vi "FaceDL.vi"(0 "Data In":T8={"positions"=[1.0, 1.0, 1.0]} caption="Données en entrée", 2 "Display State In":T6={"param"=[], "positions"=[0.0, 0.0, 0.0], "CellsI"=enum."5", "CellsIII"=enum."7", "step,ps"=100, " preset pos"=[], "event"=refnum} caption="État d'affichage en entrée", 3 "Container State":T7 caption="État du conteneur") -> (6 "Data Out":T8={"positions"=[1.0, 1.0, 1.0]} caption="Données en sortie", 7 "Display State Out":T6={"param"=[], "positions"=[0.0, 0.0, 0.0], "CellsI"=enum."5", "CellsIII"=enum."7", "step,ps"=100, " preset pos"=[], "event"=refnum} caption="État d'affichage en sortie", 8 "Action":T5)   [LabVIEW 2020, in "ControlDL.xctl"]
uses:
  ControlDL.xctl
  DataDL.ctl
  <vilib>/_xctls/Container State.ctl
  stateDL.ctl
  controls/CellsSDI.ctl
  controls/CellBoolean.ctl
  controls/CellsSDIII.ctl
  <vilib>/_xctls/Action.ctl
  controls/DLSD.ctl
  controls/DLlongVerSD.ctl
  <vilib>/_xctls/XControlSupport.lvlib
panel:
  in  "CellsI":T1
  in  "param":cluster{"min":dbl, "max":dbl, "real pos":dbl}[](array[cluster])=[{"min"=-40.0, "max"=130.0, "real pos"=-130.0}, {"min"=-900.0, "max"=100.0, "real pos"=-100.0}, {"min"=-13.0, "max"=150.0, "real pos"=-137.0}]
  in  "posI":dbl caption="posI,mm"
  in  "DLI":T2=1.0 min=0.0 max=1.0 scale format="%#_6f"
  in  "step,ps":i32
  in  "Down":bool
  in  "Up":bool
  in  "posII":dbl caption="posII, mm"
  in  "DLII":T3=1.0 min=0.0 max=1.0 scale=-0.1..1.2 scale format="%.2f"
  in  "preset pos":dbl[][](array[numeric])=[[-48.0, -24.0, 0.0, 24.0, 48.0]]
  in  "CellsIII":T4=enum."1"
  in  "posIII":dbl
  in  "DLIII":T2=1.0 min=0.0 max=1.0 scale format="%#_6f"
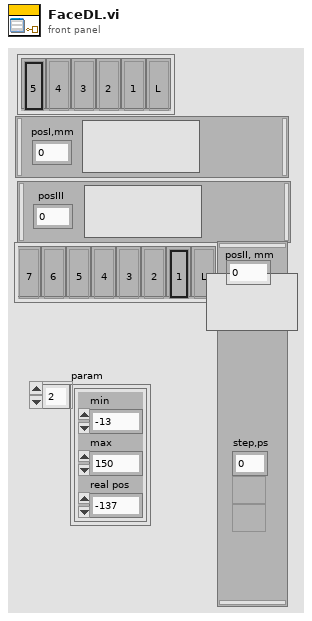
[diagram p1: front panel]
types:
  T1 = typedef "CellsSDI.ctl" = enum32{"5", "4", "3", "2", "1", "L"}
  T2 = typedef "DLSD.ctl" = dbl
  T3 = typedef "DLlongVerSD.ctl" = dbl
  T4 = typedef "CellsSDIII.ctl" = enum32{"7", "6", "5", "4", "3", "2", "1", "L"}
  T5 = typedef "XControlSupport.lvlib/Action.ctl" = cluster{"Data Changed?":bool, "State Changed?":bool, "Action Name":string}
  T6 = typedef "ControlDL.xctl/stateDL.ctl" = cluster{"param":cluster{"min":dbl, "max":dbl, "real pos":dbl}[], "positions":dbl[], "CellsI":T1, "CellsIII":T4, "step,ps":i32, " preset pos":dbl[][], "event":refnum<user-event>}
  T7 = typedef "XControlSupport.lvlib/Container State.ctl" = cluster{"Indicator?":bool, "Run Mode?":bool, " Refnum":refnum<vi>}
  T8 = typedef "ControlDL.xctl/DataDL.ctl" = cluster{"positions":dbl[]}
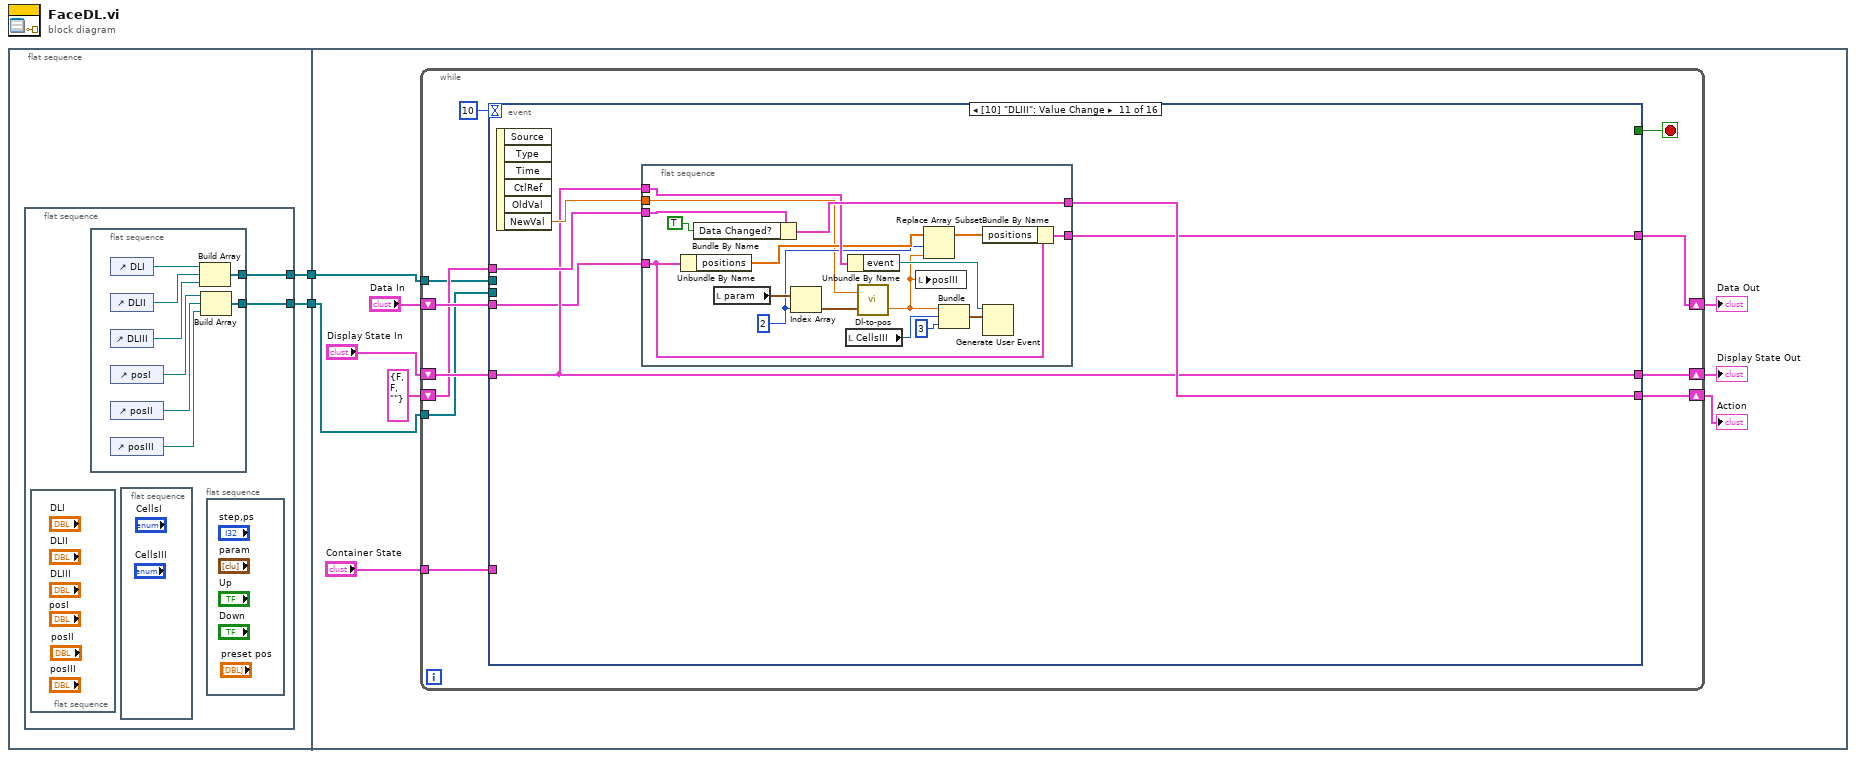
[diagram p0: block diagram]
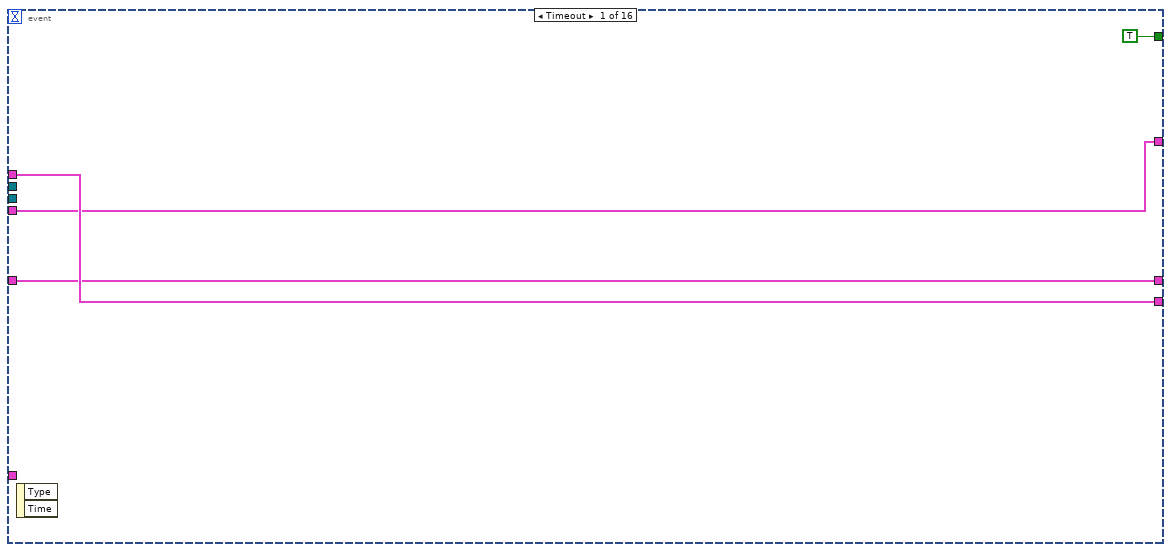
[diagram p2: hidden frame]
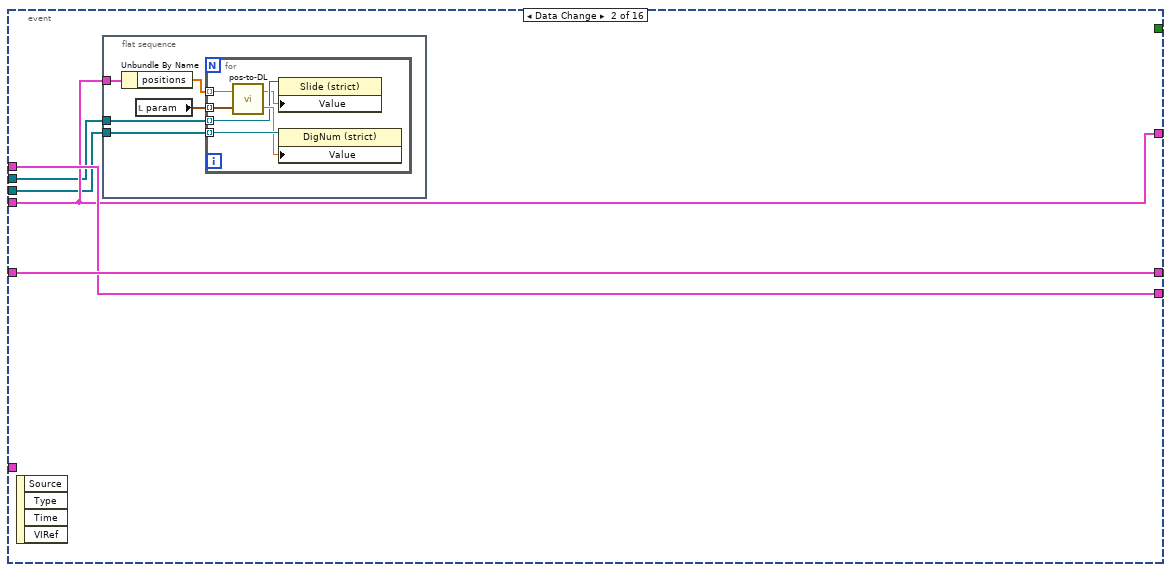
[diagram p3: hidden frame]
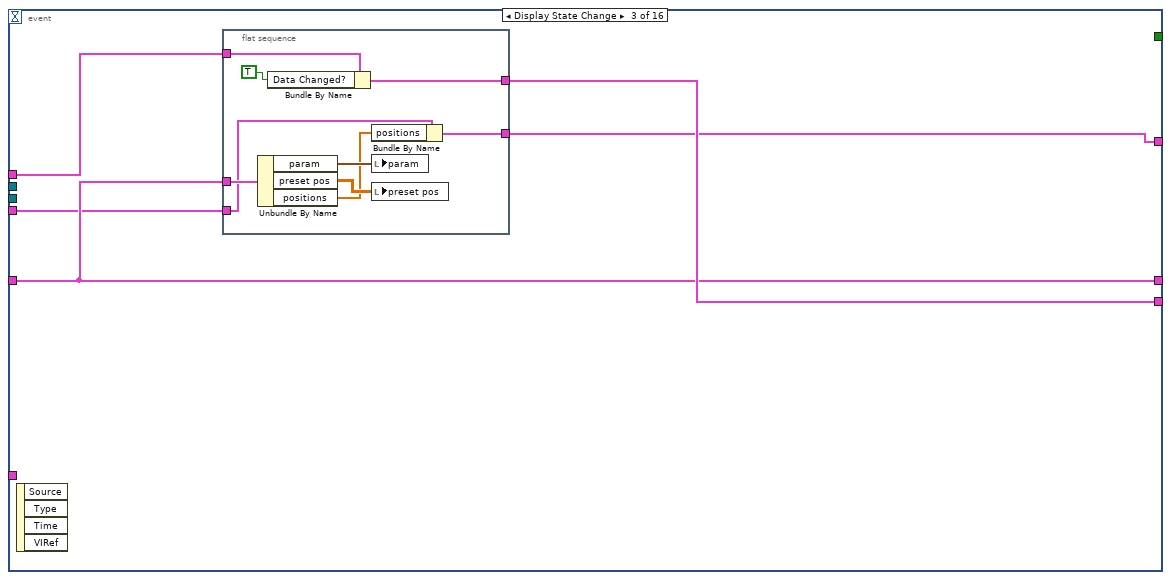
[diagram p4: hidden frame]
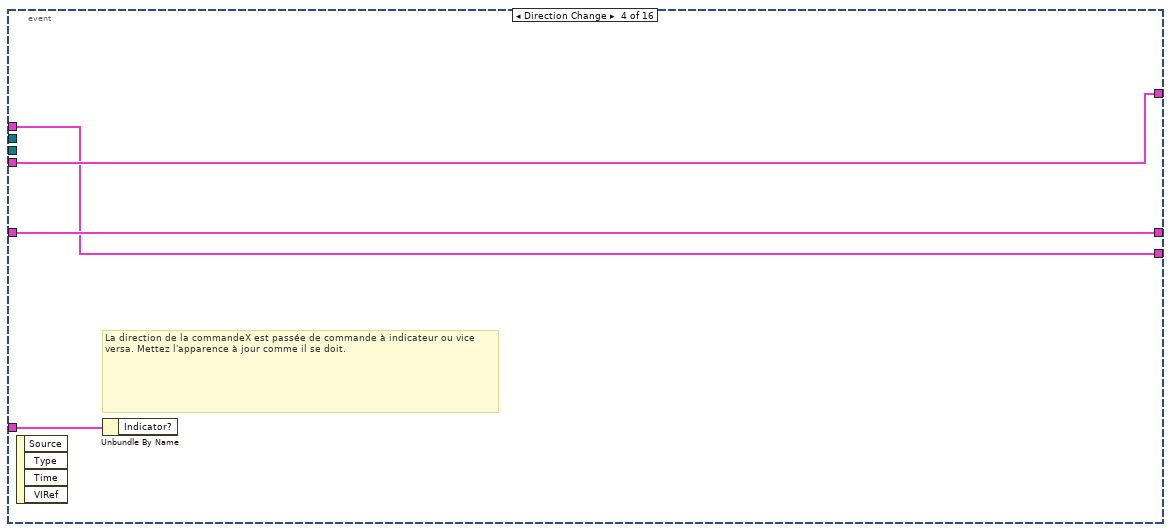
[diagram p5: hidden frame]
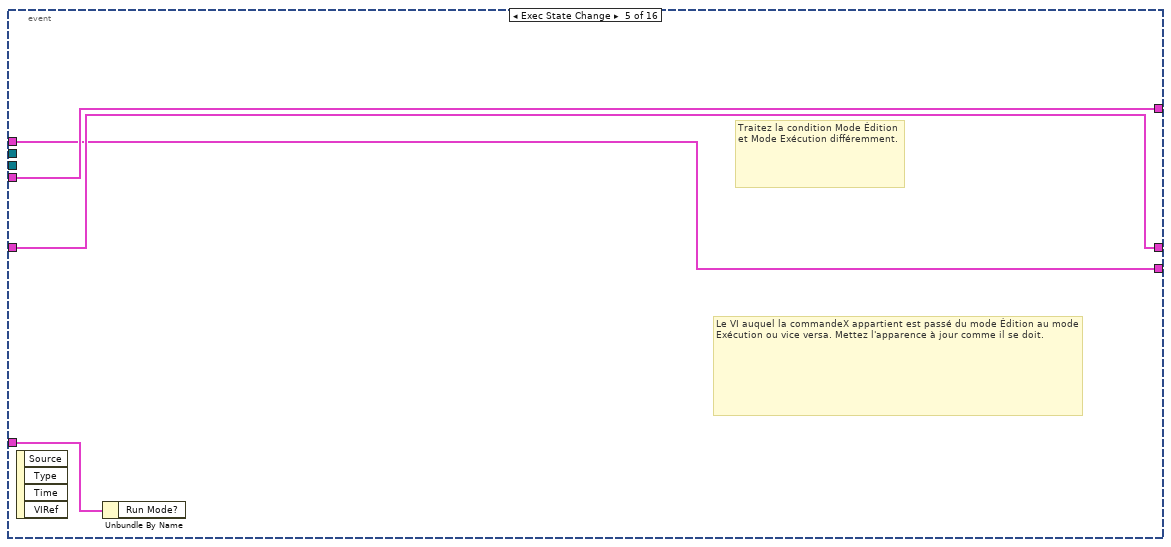
[diagram p6: hidden frame]
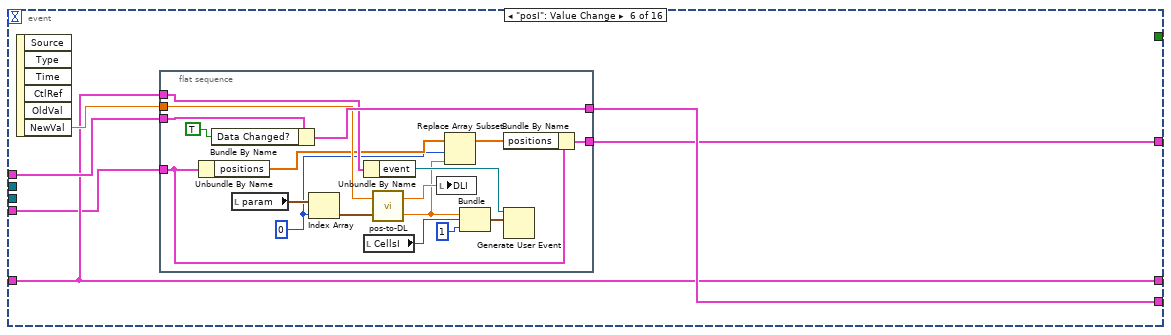
[diagram p7: hidden frame]
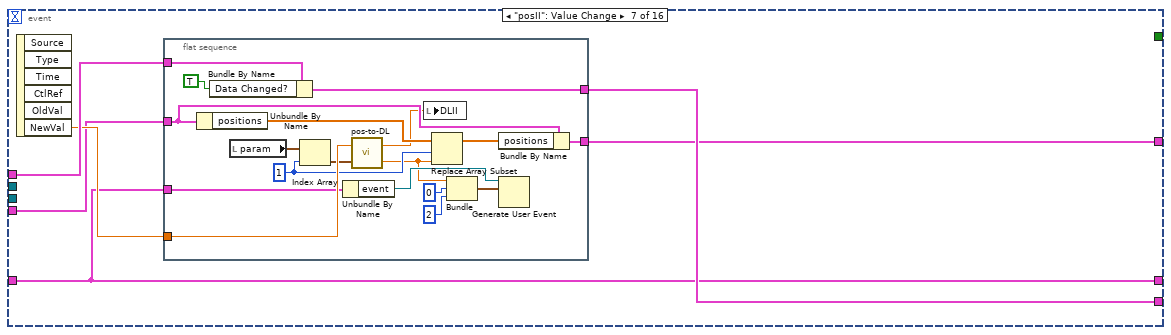
[diagram p8: hidden frame]
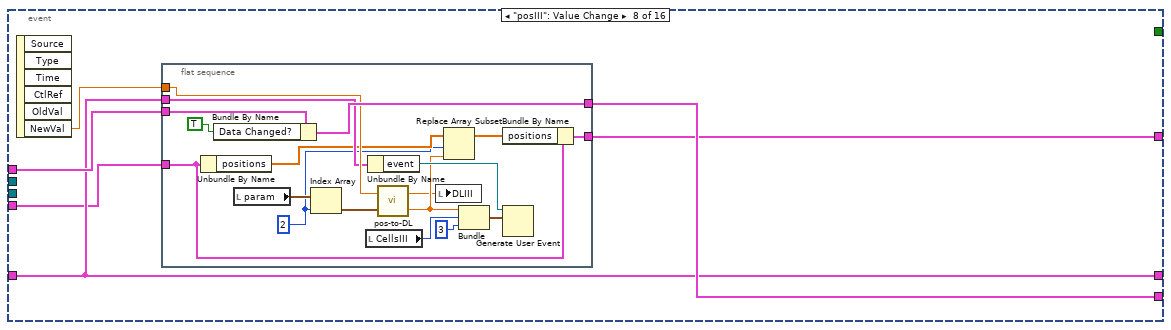
[diagram p9: hidden frame]
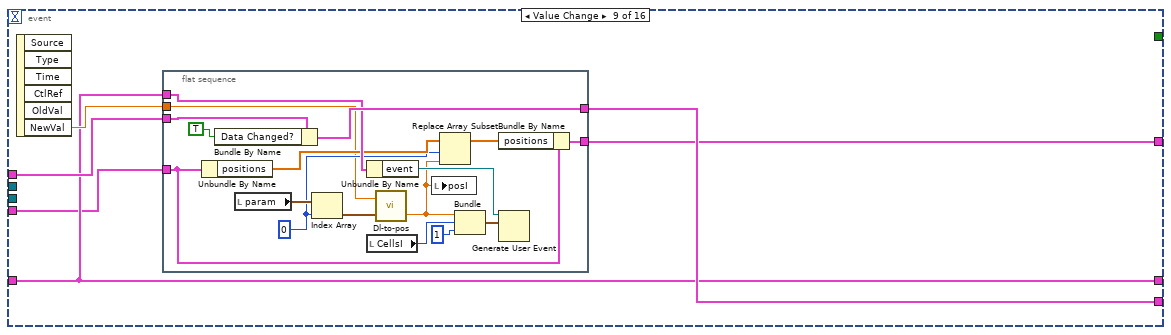
[diagram p10: hidden frame]
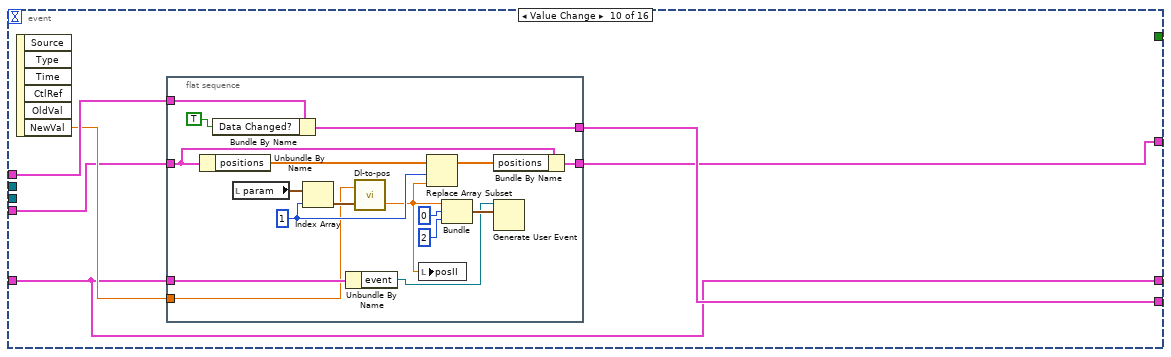
[diagram p11: hidden frame]
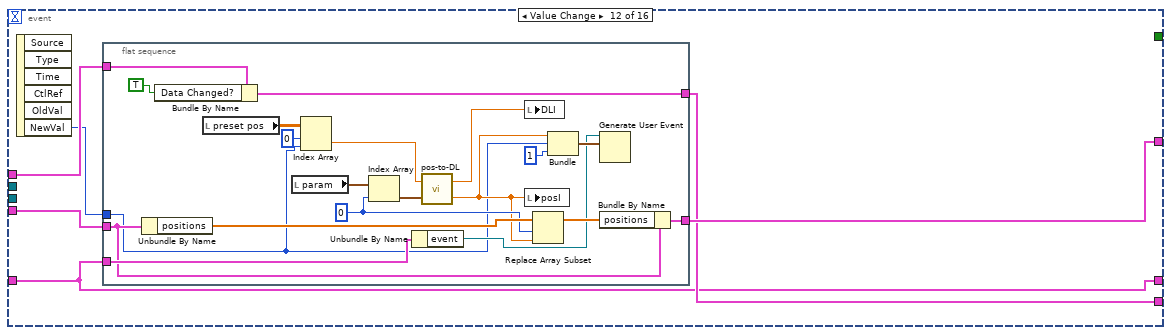
[diagram p12: hidden frame]
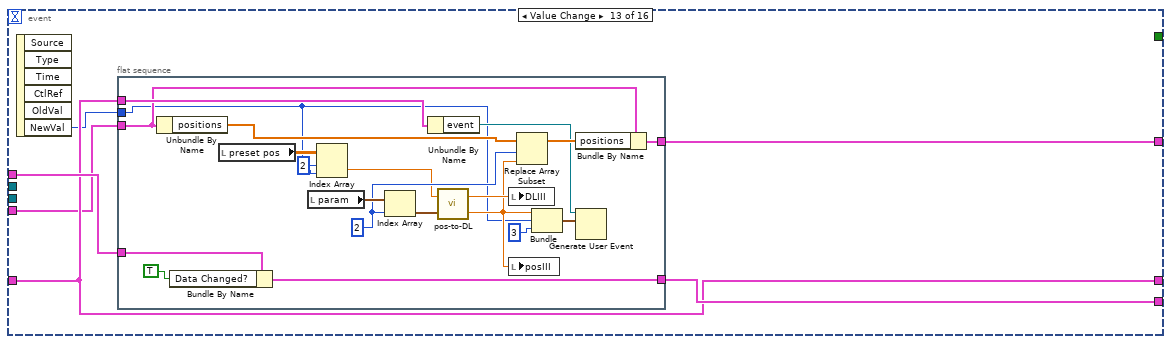
[diagram p13: hidden frame]
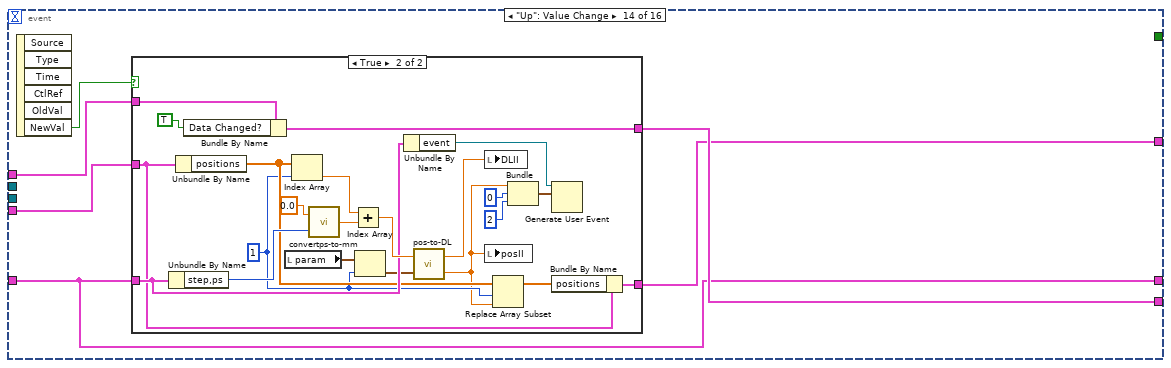
[diagram p14: hidden frame]
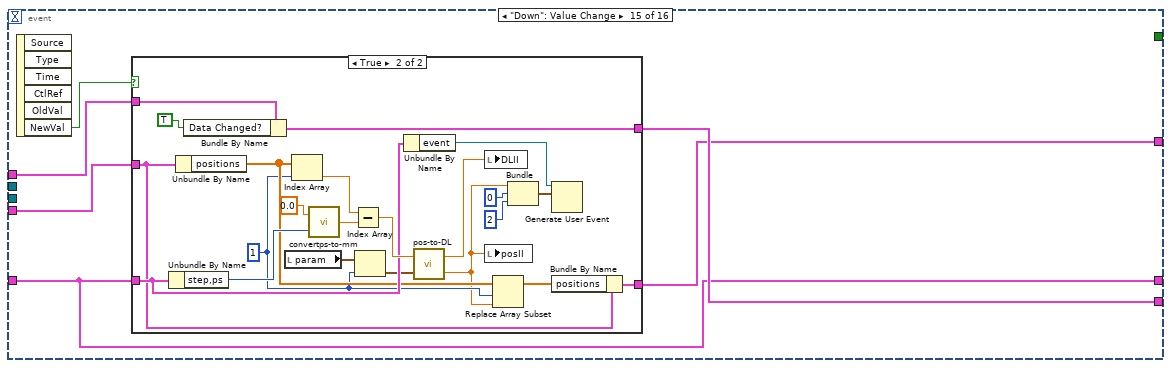
[diagram p16: hidden frame]
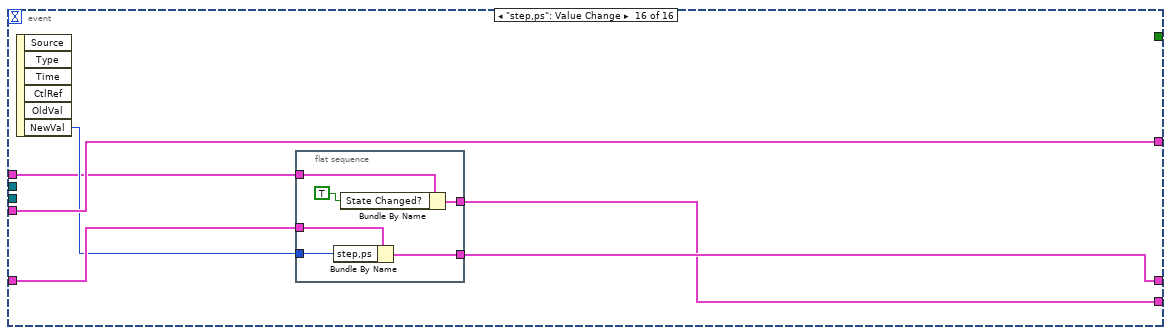
[diagram p18: hidden frame]
diagram:
  n1 = flat-sequence {
    tunnel: [w4] -> w2
    tunnel: [w3] -> w1
    tunnel: w2 -> [w16]
    tunnel: w1 -> [w15]
    frame #0 {
      n2 = flat-sequence {
        tunnel: [w6] -> w4
        tunnel: [w5] -> w3
        frame #0 {
          n3 = flat-sequence {
            frame #0 {
            }
          }
          n4 = flat-sequence {
            tunnel: [w8] -> w6
            tunnel: [w7] -> w5
            frame #0 {
              n5 = control-ref of="DLI"() -> (w11:refnum<vi>)
              n6 = control-ref of="DLII"() -> (w10:refnum<vi>)
              n7 = control-ref of="DLIII"() -> (w9:refnum<vi>)
              n8 = control-ref of="posI"() -> (w14:refnum<vi>)
              n9 = control-ref of="posII"() -> (w13:refnum<vi>)
              n10 = control-ref of="posIII"() -> (w12:refnum<vi>)
              n11 = Build Array(w11, w10, w9) -> (w7:refnum<vi>[])
              n12 = Build Array(w14, w13, w12) -> (w8:refnum<vi>[])
            }
          }
          n13 = flat-sequence {
            frame #0 {
            }
          }
          n14 = flat-sequence {
            frame #0 {
            }
          }
        }
      }
    }
    frame #1 {
      n15 = while {
        shift-right: [w33] -> w20
        shift-left: "Display State In" -> [w34]
        tunnel: "Container State" -> [w30]
        shift-right: [w28] -> w23
        shift-left: "Data In" -> [w29]
        shift-right: [w26] -> w19
        shift-left: T5 {"Data Changed?"=FALSE, "State Changed?"=FALSE, "Action Name"=""} ("Action") -> [w27]
        tunnel: w16 -> [w25]
        tunnel: w15 -> [w24]
        stop <- w32 stop-if-true
        n16 = event shown="[10] \"DLIII\": Value Change" {
          selector: _ -> [_ _ _ _ _ _ _ _ _ _ _ _ _ _ _ _]
          dyn-events: _ -> [_ _ _ _ _ _ _ _ _ _ _ _ _ _ _ _]
          timeout: 10 -> [_ _ _ _ _ _ _ _ _ _ _ _ _ _ _ _]
          tunnel: w34 -> [w36 w43 w57 w71 w75 w78 w102 w126 w150 w173 w196 w220 w246 w272 w302 w334]
          tunnel: [w36 w43 w57 w71 w75 w78 w102 w126 w150 w173 w196 w220 w246 w272 w302 w333] -> w33
          tunnel: [TRUE _ _ _ _ _ _ _ _ _ _ _ _ _ _ _] -> w32
          tunnel: w30 -> [_ _ _ w72 w76 _ _ _ _ _ _ _ _ _ _ _]
          tunnel: w29 -> [w35 w41 w56 w70 w74 w77 w101 w125 w149 w172 w195 w218 w244 w271 w301 w335]
          tunnel: [w35 w41 w55 w70 w74 w80 w104 w128 w152 w175 w198 w223 w249 w273 w303 w335] -> w28
          tunnel: [w37 w42 w58 w69 w73 w81 w105 w129 w153 w176 w199 w221 w247 w274 w304 w330] -> w26
          tunnel: w27 -> [w37 w42 w59 w69 w73 w82 w106 w130 w154 w177 w200 w222 w248 w275 w305 w331]
          tunnel: w25 -> [_ w40 _ _ _ _ _ _ _ _ _ _ _ _ _ _]
          tunnel: w24 -> [_ w39 _ _ _ _ _ _ _ _ _ _ _ _ _ _]
          event Timeout {
            n17 = event-data() -> ()  [unwired: 1 in, 2 out]
          }
          event Data Change {
            n18 = event-data() -> ()  [unwired: 1 in, 4 out]
            n19 = flat-sequence {
              tunnel: w41 -> [w48]
              tunnel: w40 -> [w45]
              tunnel: w39 -> [w44]
              frame #0 {
                n20 = Unbundle By Name(w48) -> ("positions"=w47:dbl[])
                n21 = local read "param"() -> (w46:cluster{"min":dbl, "max":dbl, "real pos":dbl}[])
                n22 = for {
                  tunnel: w47 -> [w54] mode=indexing
                  tunnel: w46 -> [w53] mode=indexing
                  tunnel: w45 -> [w52] mode=indexing
                  tunnel: w44 -> [w50] mode=indexing
                  n23 = call "pos-to-DL.vi"("DL param"=w53, "pos, mm"=w54) -> ("pos, mm"=w51:dbl, "DL pos"=w49:dbl)
                  n24 = property class="Slide (strict)"(reference=w50, "Value"=w49) -> ()  [unwired: 1 in, 2 out]
                  n25 = property class="DigNum (strict)"(reference=w52, "Value"=w51) -> ()  [unwired: 1 in, 2 out]
                }
              }
            }
          }
          event Display State Change {
            n26 = event-data() -> ()  [unwired: 1 in, 4 out]
            n27 = flat-sequence {
              tunnel: w59 -> [w68]
              tunnel: [w67] -> w58
              tunnel: w57 -> [w65]
              tunnel: w56 -> [w62]
              tunnel: [w61] -> w55
              frame #0 {
                n28 = Unbundle By Name(w65) -> ("param"=w63:cluster{"min":dbl, "max":dbl, "real pos":dbl}[], "preset pos"=w64:dbl[][], "positions"=w60:dbl[])
                n29 = Bundle By Name(cluster=w68, "Data Changed?"=TRUE) -> (w67:T5)
                n30 = Bundle By Name(cluster=w62, "positions"=w60) -> (w61:T8)
                n31 = local write "param"(w63) -> ()
                n32 = local write "preset pos"(w64) -> ()
              }
            }
          }
          event Direction Change {
            # "La direction de la commandeX est passée de commande à indicateur ou vice versa. Mettez l'apparence à jour comme il se doit."
            n33 = event-data() -> ()  [unwired: 1 in, 4 out]
            n34 = Unbundle By Name(w72) -> ()  [unwired: 1 out]
          }
          event Exec State Change {
            # "Le VI auquel la commandeX appartient est passé du mode Édition au mode Exécution ou vice versa. Mettez l'apparence à jour comme il se doit."
            # "Traitez la condition Mode Édition et Mode Exécution différemment."
            n35 = event-data() -> ()  [unwired: 1 in, 4 out]
            n36 = Unbundle By Name(w76) -> ()  [unwired: 1 out]
          }
          event "posI": Value Change {
            n37 = event-data() -> ("NewVal"=w79:dbl)  [unwired: 1 in, 5 out]
            n38 = flat-sequence {
              tunnel: w82 -> [w100]
              tunnel: [w99] -> w81
              tunnel: [w97] -> w80
              tunnel: w79 -> [w96]
              tunnel: w78 -> [w95]
              tunnel: w77 -> [w92]
              frame #0 {
                w89 = 0 ("index")
                n39 = Unbundle By Name(w92) -> ("positions"=w91:dbl[])
                n40 = Bundle By Name(cluster=w100, "Data Changed?"=TRUE ("State Changed?")) -> (w99:T5)
                n41 = local read "param"() -> (w94:cluster{"min":dbl, "max":dbl, "real pos":dbl}[])
                n42 = Index Array(array=w94, index=w89) -> (element=w93:cluster{"min":dbl, "max":dbl, "real pos":dbl})
                n43 = Unbundle By Name(w95) -> ("event"=w85:refnum<user-event>)
                n44 = local read "CellsI"() -> (w87:T1)
                n45 = call "pos-to-DL.vi"("DL param"=w93, "pos, mm"=w96) -> ("pos, mm"=w83:dbl, "DL pos"=w84:dbl)
                n46 = local write "DLI"(w84) -> ()
                n47 = Replace Array Subset(array=w91, new element=w83, index=w89) -> (w90:dbl[])
                n48 = Bundle("pos, mm"=w83, "CellsI"=w87, 1) -> (w88:cluster{"pos, mm":dbl, "CellsI":T1, i32})  [unwired: 1 in]
                n49 = Bundle By Name(cluster=w92, "positions"=w90) -> (w97:T8)
                n50 = Generate User Event(user event=w85, event data cluster=w88) -> ()  [unwired: 2 in, 2 out]
              }
            }
          }
          event "posII": Value Change {
            n51 = event-data() -> ("NewVal"=w103:dbl)  [unwired: 1 in, 5 out]
            n52 = flat-sequence {
              tunnel: w106 -> [w124]
              tunnel: [w123] -> w105
              tunnel: [w121] -> w104
              tunnel: w103 -> [w120]
              tunnel: w102 -> [w119]
              tunnel: w101 -> [w116]
              frame #0 {
                w113 = 1 ("index")
                n53 = Unbundle By Name(w116) -> ("positions"=w115:dbl[])
                n54 = Bundle By Name(cluster=w124, "Data Changed?"=TRUE ("State Changed?")) -> (w123:T5)
                n55 = local read "param"() -> (w118:cluster{"min":dbl, "max":dbl, "real pos":dbl}[])
                n56 = Index Array(array=w118, index=w113) -> (element=w117:cluster{"min":dbl, "max":dbl, "real pos":dbl})
                n57 = Unbundle By Name(w119) -> ("event"=w110:refnum<user-event>)
                n58 = call "pos-to-DL.vi"("DL param"=w117, "pos, mm"=w120) -> ("pos, mm"=w109:dbl, "DL pos"=w108:dbl)
                n59 = local write "DLII"(w108) -> ()
                n60 = Replace Array Subset(array=w115, new element=w109, index=w113) -> (w114:dbl[])
                n61 = Bundle("pos, mm"=w109, 0, 2) -> (w107:cluster{"pos, mm":dbl, i32, i32})  [unwired: 1 in]
                n62 = Bundle By Name(cluster=w116, "positions"=w114) -> (w121:T8)
                n63 = Generate User Event(user event=w110, event data cluster=w107) -> ()  [unwired: 2 in, 2 out]
              }
            }
          }
          event "posIII": Value Change {
            n64 = event-data() -> ("NewVal"=w127:dbl)  [unwired: 1 in, 5 out]
            n65 = flat-sequence {
              tunnel: w130 -> [w148]
              tunnel: [w147] -> w129
              tunnel: [w145] -> w128
              tunnel: w127 -> [w144]
              tunnel: w126 -> [w143]
              tunnel: w125 -> [w140]
              frame #0 {
                w137 = 2 ("index")
                n66 = Unbundle By Name(w140) -> ("positions"=w139:dbl[])
                n67 = Bundle By Name(cluster=w148, "Data Changed?"=TRUE ("State Changed?")) -> (w147:T5)
                n68 = local read "param"() -> (w142:cluster{"min":dbl, "max":dbl, "real pos":dbl}[])
                n69 = Index Array(array=w142, index=w137) -> (element=w141:cluster{"min":dbl, "max":dbl, "real pos":dbl})
                n70 = local read "CellsIII"() -> (w135:T4)
                n71 = Unbundle By Name(w143) -> ("event"=w133:refnum<user-event>)
                n72 = call "pos-to-DL.vi"("DL param"=w141, "pos, mm"=w144) -> ("pos, mm"=w132:dbl, "DL pos"=w131:dbl)
                n73 = local write "DLIII"(w131) -> ()
                n74 = Replace Array Subset(array=w139, new element=w132, index=w137) -> (w138:dbl[])
                n75 = Bundle("pos, mm"=w132, "CellsIII"=w135, 3) -> (w136:cluster{"pos, mm":dbl, "CellsIII":T4, i32})  [unwired: 1 in]
                n76 = Bundle By Name(cluster=w140, "positions"=w138) -> (w145:T8)
                n77 = Generate User Event(user event=w133, event data cluster=w136) -> ()  [unwired: 2 in, 2 out]
              }
            }
          }
          event Value Change {
            n78 = event-data() -> ("NewVal"=w151:T2)  [unwired: 1 in, 5 out]
            n79 = flat-sequence {
              tunnel: w154 -> [w171]
              tunnel: [w170] -> w153
              tunnel: [w168] -> w152
              tunnel: w151 -> [w159]
              tunnel: w150 -> [w167]
              tunnel: w149 -> [w165]
              frame #0 {
                w162 = 0 ("index")
                n80 = Unbundle By Name(w165) -> ("positions"=w164:dbl[])
                n81 = Bundle By Name(cluster=w171, "Data Changed?"=TRUE ("State Changed?")) -> (w170:T5)
                n82 = local read "param"() -> (w166:cluster{"min":dbl, "max":dbl, "real pos":dbl}[])
                n83 = Index Array(array=w166, index=w162) -> (element=w160:cluster{"min":dbl, "max":dbl, "real pos":dbl})
                n84 = Unbundle By Name(w167) -> ("event"=w156:refnum<user-event>)
                n85 = local read "CellsI"() -> (w161:T1)
                n86 = call "Dl-to-pos.vi"("DL param"=w160, "DL_pos"=w159) -> ("pos, mm"=w155:dbl)  [unwired: 1 out]
                n87 = local write "posI"(w155) -> ()
                n88 = Replace Array Subset(array=w164, new element=w155, index=w162) -> (w163:dbl[])
                n89 = Bundle("pos, mm"=w155, "CellsI"=w161, 1) -> (w158:cluster{"pos, mm":dbl, "CellsI":T1, i32})  [unwired: 1 in]
                n90 = Bundle By Name(cluster=w165, "positions"=w163) -> (w168:T8)
                n91 = Generate User Event(user event=w156, event data cluster=w158) -> ()  [unwired: 2 in, 2 out]
              }
            }
          }
          event Value Change {
            n92 = event-data() -> ("NewVal"=w174:T3)  [unwired: 1 in, 5 out]
            n93 = flat-sequence {
              tunnel: w177 -> [w194]
              tunnel: [w193] -> w176
              tunnel: [w191] -> w175
              tunnel: w174 -> [w183]
              tunnel: w173 -> [w190]
              tunnel: w172 -> [w188]
              frame #0 {
                w185 = 1 ("index")
                n94 = Unbundle By Name(w188) -> ("positions"=w187:dbl[])
                n95 = Bundle By Name(cluster=w194, "Data Changed?"=TRUE ("State Changed?")) -> (w193:T5)
                n96 = local read "param"() -> (w189:cluster{"min":dbl, "max":dbl, "real pos":dbl}[])
                n97 = Index Array(array=w189, index=w185) -> (element=w184:cluster{"min":dbl, "max":dbl, "real pos":dbl})
                n98 = Unbundle By Name(w190) -> ("event"=w179:refnum<user-event>)
                n99 = call "Dl-to-pos.vi"("DL param"=w184, "DL_pos"=w183) -> ("pos, mm"=w178:dbl)  [unwired: 1 out]
                n100 = local write "posII"(w178) -> ()
                n101 = Replace Array Subset(array=w187, new element=w178, index=w185) -> (w186:dbl[])
                n102 = Bundle("pos, mm"=w178, 0, 2) -> (w181:cluster{"pos, mm":dbl, i32, i32})  [unwired: 1 in]
                n103 = Bundle By Name(cluster=w188, "positions"=w186) -> (w191:T8)
                n104 = Generate User Event(user event=w179, event data cluster=w181) -> ()  [unwired: 2 in, 2 out]
              }
            }
          }
          event Value Change {
            n105 = event-data() -> ("NewVal"=w197:T2)  [unwired: 1 in, 5 out]
            n106 = flat-sequence {
              tunnel: w200 -> [w217]
              tunnel: [w216] -> w199
              tunnel: [w214] -> w198
              tunnel: w197 -> [w206]
              tunnel: w196 -> [w213]
              tunnel: w195 -> [w211]
              frame #0 {
                w208 = 2 ("index")
                n107 = Unbundle By Name(w211) -> ("positions"=w210:dbl[])
                n108 = Bundle By Name(cluster=w217, "Data Changed?"=TRUE ("State Changed?")) -> (w216:T5)
                n109 = local read "param"() -> (w212:cluster{"min":dbl, "max":dbl, "real pos":dbl}[])
                n110 = Index Array(array=w212, index=w208) -> (element=w207:cluster{"min":dbl, "max":dbl, "real pos":dbl})
                n111 = local read "CellsIII"() -> (w205:T4)
                n112 = Unbundle By Name(w213) -> ("event"=w202:refnum<user-event>)
                n113 = call "Dl-to-pos.vi"("DL param"=w207, "DL_pos"=w206) -> ("pos, mm"=w201:dbl)  [unwired: 1 out]
                n114 = local write "posIII"(w201) -> ()
                n115 = Replace Array Subset(array=w210, new element=w201, index=w208) -> (w209:dbl[])
                n116 = Bundle("pos, mm"=w201, "CellsIII"=w205, 3) -> (w204:cluster{"pos, mm":dbl, "CellsIII":T4, i32})  [unwired: 1 in]
                n117 = Bundle By Name(cluster=w211, "positions"=w209) -> (w214:T8)
                n118 = Generate User Event(user event=w202, event data cluster=w204) -> ()  [unwired: 2 in, 2 out]
              }
            }
          }
          event Value Change {
            n119 = event-data() -> ("NewVal"=w219:T1)  [unwired: 1 in, 5 out]
            n120 = flat-sequence {
              tunnel: [w243] -> w223
              tunnel: w222 -> [w242]
              tunnel: [w241] -> w221
              tunnel: w220 -> [w238]
              tunnel: w219 -> [w226]
              tunnel: w218 -> [w234]
              frame #0 {
                w231 = 0 ("index")
                n121 = Unbundle By Name(w234) -> ("positions"=w233:dbl[])
                n122 = Bundle By Name(cluster=w242, "Data Changed?"=TRUE) -> (w241:T5)
                n123 = local read "preset pos"() -> (w230:dbl[][])
                n124 = local read "param"() -> (w237:cluster{"min":dbl, "max":dbl, "real pos":dbl}[])
                n125 = Index Array(array=w230, index (row)=0 ("disabled index (row)"), index (col)=w226) -> (element=w224:dbl)
                n126 = Index Array(array=w237, index=w231) -> (element=w236:cluster{"min":dbl, "max":dbl, "real pos":dbl})
                n127 = Unbundle By Name(w238) -> ("event"=w227:refnum<user-event>)
                n128 = call "pos-to-DL.vi"("DL param"=w236, "pos, mm"=w224) -> ("pos, mm"=w229:dbl, "DL pos"=w239:dbl)
                n129 = local write "DLI"(w239) -> ()
                n130 = local write "posI"(w229) -> ()
                n131 = Replace Array Subset(array=w233, new element=w229, index=w231) -> (w232:dbl[])
                n132 = Bundle("pos, mm"=w229, "NewVal"=w226, 1) -> (w235:cluster{"pos, mm":dbl, "NewVal":T1, i32})  [unwired: 1 in]
                n133 = Generate User Event(user event=w227, event data cluster=w235) -> ()  [unwired: 2 in, 2 out]
                n134 = Bundle By Name(cluster=w234, "positions"=w232) -> (w243:T8)
              }
            }
          }
          event Value Change {
            n135 = event-data() -> ("NewVal"=w245:T4)  [unwired: 1 in, 5 out]
            n136 = flat-sequence {
              tunnel: [w269] -> w249
              tunnel: w248 -> [w268]
              tunnel: [w267] -> w247
              tunnel: w246 -> [w264]
              tunnel: w245 -> [w252]
              tunnel: w244 -> [w260]
              frame #0 {
                w257 = 2 ("index")
                n137 = Unbundle By Name(w260) -> ("positions"=w259:dbl[])
                n138 = Bundle By Name(cluster=w268, "Data Changed?"=TRUE) -> (w267:T5)
                n139 = local read "preset pos"() -> (w256:dbl[][])
                n140 = local read "param"() -> (w263:cluster{"min":dbl, "max":dbl, "real pos":dbl}[])
                n141 = Index Array(array=w256, index (row)=2 ("disabled index (row)"), index (col)=w252) -> (element=w250:dbl)
                n142 = Index Array(array=w263, index=w257) -> (element=w262:cluster{"min":dbl, "max":dbl, "real pos":dbl})
                n143 = Unbundle By Name(w264) -> ("event"=w253:refnum<user-event>)
                n144 = call "pos-to-DL.vi"("DL param"=w262, "pos, mm"=w250) -> ("pos, mm"=w255:dbl, "DL pos"=w265:dbl)
                n145 = local write "DLIII"(w265) -> ()
                n146 = local write "posIII"(w255) -> ()
                n147 = Replace Array Subset(array=w259, new element=w255, index=w257) -> (w258:dbl[])
                n148 = Bundle("pos, mm"=w255, "NewVal"=w252, 3) -> (w261:cluster{"pos, mm":dbl, "NewVal":T4, i32})  [unwired: 1 in]
                n149 = Bundle By Name(cluster=w260, "positions"=w258) -> (w269:T8)
                n150 = Generate User Event(user event=w253, event data cluster=w261) -> ()  [unwired: 2 in, 2 out]
              }
            }
          }
          event "Up": Value Change {
            n151 = event-data() -> ("NewVal"=w270:bool)  [unwired: 1 in, 5 out]
            n152 = case shown="True" w270 {
              tunnel: w275 -> [w276 w299]
              tunnel: [w276 w298] -> w274
              tunnel: [w277 w296] -> w273
              tunnel: w272 -> [_ w291]
              tunnel: w271 -> [w277 w287]
              frame False {
              }
              frame True {
                w282 = 1 ("index")
                n153 = Unbundle By Name(w291) -> ("step,ps"=w290:i32)
                n154 = Unbundle By Name(w287) -> ("positions"=w285:dbl[])
                n155 = Bundle By Name(cluster=w299, "Data Changed?"=TRUE ("State Changed?")) -> (w298:T5)
                n156 = local read "param"() -> (w289:cluster{"min":dbl, "max":dbl, "real pos":dbl}[])
                n157 = Index Array(array=w285, index=w282) -> (element=w284:dbl)
                n158 = call "convertps-to-mm.vi"("ps"=w290, "Real zero"=0.0) -> ("mm"=w293:dbl)
                n159 = Add(x=w284, y=w293) -> (x+y=w292:dbl)
                n160 = Index Array(array=w289, index=w282) -> (element=w288:cluster{"min":dbl, "max":dbl, "real pos":dbl})
                n161 = Unbundle By Name(w291) -> ("event"=w278:refnum<user-event>)
                n162 = call "pos-to-DL.vi"("DL param"=w288, "pos, mm"=w292) -> ("pos, mm"=w280:dbl, "DL pos"=w295:dbl)
                n163 = local write "DLII"(w295) -> ()
                n164 = local write "posII"(w280) -> ()
                n165 = Replace Array Subset(array=w285, new element=w280, index=w282) -> (w286:dbl[])
                n166 = Bundle("pos, mm"=w280, "index"=0, 2) -> (w279:cluster{"pos, mm":dbl, "index":i32, i32})  [unwired: 1 in]
                n167 = Generate User Event(user event=w278, event data cluster=w279) -> ()  [unwired: 2 in, 2 out]
                n168 = Bundle By Name(cluster=w287, "positions"=w286) -> (w296:T8)
              }
            }
          }
          event "Down": Value Change {
            n169 = event-data() -> ("NewVal"=w300:bool)  [unwired: 1 in, 5 out]
            n170 = case shown="True" w300 {
              tunnel: w305 -> [w306 w329]
              tunnel: [w306 w328] -> w304
              tunnel: [w307 w326] -> w303
              tunnel: w302 -> [_ w321]
              tunnel: w301 -> [w307 w317]
              frame False {
              }
              frame True {
                w312 = 1 ("index")
                n171 = Unbundle By Name(w321) -> ("step,ps"=w320:i32)
                n172 = Unbundle By Name(w317) -> ("positions"=w315:dbl[])
                n173 = Bundle By Name(cluster=w329, "Data Changed?"=TRUE ("State Changed?")) -> (w328:T5)
                n174 = local read "param"() -> (w319:cluster{"min":dbl, "max":dbl, "real pos":dbl}[])
                n175 = Index Array(array=w315, index=w312) -> (element=w314:dbl)
                n176 = call "convertps-to-mm.vi"("ps"=w320, "Real zero"=0.0) -> ("mm"=w323:dbl)
                n177 = Subtract(x=w314, y=w323) -> (x-y=w322:dbl)
                n178 = Index Array(array=w319, index=w312) -> (element=w318:cluster{"min":dbl, "max":dbl, "real pos":dbl})
                n179 = Unbundle By Name(w321) -> ("event"=w308:refnum<user-event>)
                n180 = call "pos-to-DL.vi"("DL param"=w318, "pos, mm"=w322) -> ("pos, mm"=w310:dbl, "DL pos"=w325:dbl)
                n181 = local write "DLII"(w325) -> ()
                n182 = local write "posII"(w310) -> ()
                n183 = Replace Array Subset(array=w315, new element=w310, index=w312) -> (w316:dbl[])
                n184 = Bundle("pos, mm"=w310, "index"=0, 2) -> (w309:cluster{"pos, mm":dbl, "index":i32, i32})  [unwired: 1 in]
                n185 = Generate User Event(user event=w308, event data cluster=w309) -> ()  [unwired: 2 in, 2 out]
                n186 = Bundle By Name(cluster=w317, "positions"=w316) -> (w326:T8)
              }
            }
          }
          event "step,ps": Value Change {
            n187 = event-data() -> ("NewVal"=w332:i32)  [unwired: 1 in, 5 out]
            n188 = flat-sequence {
              tunnel: w334 -> [w341]
              tunnel: [w340] -> w333
              tunnel: w332 -> [w339]
              tunnel: w331 -> [w338]
              tunnel: [w337] -> w330
              frame #0 {
                n189 = Bundle By Name(cluster=w341, "step,ps"=w339) -> (w340:T6)
                n190 = Bundle By Name(cluster=w338, "State Changed?"=TRUE) -> (w337:T5)
              }
            }
          }
        }
      }
      "Display State Out" <- w20
      "Data Out" <- w23
      "Action" <- w19
    }
  }
